vi "main.vi"() -> ()   [LabVIEW 2016]
uses:
  Common_FPGA_HealthAndStatus/DataTypes/HealthAndStatusSettings.ctl
  Common_FPGA_Modbus/DataTypes/ModbusPortSettings.ctl
  Common_FPGA_Timestamp/DataTypes/TimestampSettings.ctl
  <vilib>/Platform/TimedLoop/XDataNode/timing_clust.ctl
  <vilib>/Platform/TimedLoop/XDataNode/nitl_modes.ctl
  <vilib>/Platform/TimedLoop/XDataNode/wakeup.ctl
  <vilib>/rvi/Emulation/niFpgaGetClockAttributes.vi
  <vilib>/rvi/Emulation/niFpgaSctlEmulationGetInTimedLoop.vi
  <vilib>/rvi/Emulation/niFpgaEmulationReportErrorSimple.vi
  <vilib>/rvi/eio/common/nirviEmuTemplateMethod_errors.vi
  <vilib>/rvi/Emulation/niFpgaCriticalErrorInLSC.vi
  <vilib>/rvi/Emulation/niFpgaEmulationIsFPGAContextNoSignature.vi
  <vilib>/rvi/DataTransferAndStorage/Container/Common/niFpgaContainerGetUniqueNameForEmu.vi
  <vilib>/rvi/Memory/Memory_Emulation/niFpgaMemoryEmulationCacheClearOnFirstRun.vi
  <vilib>/rvi/Memory/Memory_Emulation/nirvimemoryEmulationManagerCache_MakeExclusive.vi
  <vilib>/rvi/Memory/Memory_Emulation/niFpgaMemoryEmulationValidateCache.vi
  <vilib>/rvi/Memory/Memory_Emulation/nirvimemoryEmulationManagerCache_InsertValue.vi
  <vilib>/Utility/error.llb/Clear Errors.vi
  <vilib>/rvi/Memory/Memory_Emulation/nirvimemoryEmulationManagerCache_ReleaseExclusive.vi
  <vilib>/rvi/Memory/Memory_Emulation/nirvimemoryEmulationManagerCache_GetValue.vi
  <vilib>/rvi/Memory/Memory_Emulation/nirvimemoryEmulationManagerCache_SetValue.vi
  <vilib>/rvi/Emulation/niFpgaProcessEmulError.vi
  <vilib>/rvi/interface/RandomDataEmulation/niFpgaRandomDataHandleErrors.vi
  <vilib>/rvi/errors/niFpgaSetErrorForExecOnDevCompSimple.vi
  <vilib>/rvi/eio/common/nirviEmuReportErrorAndStop.vi
  <vilib>/rvi/FIFO/Fifo_Resource/nirvififoEmulationSetSize.vi
  <vilib>/rvi/FIFO/Fifo_Resource/nirviFifoEmulationQueueMgr.vi
  <instcachedir>/0/nirviFifoEmulationQueueMgr_E5CAEC123FF24DC58D834DCA3CDAA9B5.lvgen/nirviFifoEmulationQueueMgr_E5CAEC123FF24DC58D834DCA3CDAA9B5_002.vi
  <vilib>/rvi/FIFO/Fifo_Resource/nirvififoEmulationDetermineInputValidOut.vi
  <vilib>/rvi/FIFO/Fifo_Resource/nirvififoEmulationCreateLock.vi
  <vilib>/rvi/FIFO/Fifo_Resource/nirvififoEmulationObtainLock.vi
  <vilib>/rvi/FIFO/Fifo_Resource/nirvififoEmulationReleaseLock.vi
  <vilib>/rvi/occurrence/nirviWaitOnOccurrenceBase.vi
  <vilib>/rvi/errors/nirviReportUnexpectedCaseInternalError.vi
  <vilib>/rvi/errors/nirviReportUnexpectedCaseInternalError (U32).vi
  <vilib>/eio/EIOMethodNode/EIOMethodNode.xnode
  <vilib>/rvi/DataTransferAndStorage/Container/XNode/niFpgaContainer.xnode
  <vilib>/rvi/DataTransferAndStorage/Register/Emulation/niFpgaRegisterEmulation.vi
  <vilib>/Platform/TimedLoop/XDataNode/XDataNode.xnode
  <vilib>/rvi/interface/RandomDataEmulation/nirviRandomDataFpgaReadWriteTemplate.vi
  <vilib>/rvi/FIFO/Fifo_Resource/nirvififoEmulationWrite.vi
  Common_FPGA_HealthAndStatus/FPGAHealthAndStatus.lvlib
  Common_FPGA_Modbus/FPGAModbus.lvlib
  Common_FPGA_Timestamp/FPGATimestamp.lvlib
  <vilib>/Platform/TimedLoop/XDataNode/XDNodeRunTimeDep.lvlib
panel:
  in  "Trigger":bool
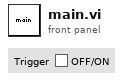
[diagram p1: front panel]
types:
  T1 = typedef "FPGATimestamp.lvlib/TimestampSettings.ctl" = cluster{"TimeRegister":refnum<k21>, "TimeSource":refnum<k21>, "IterationsPerMicrosecond":i16, "UpdateFIFO":refnum<k21>}
  T2 = typedef "FPGAModbus.lvlib/ModbusPortSettings.ctl" = cluster{"TxPort":refnum<k21>, "TxDataFIFO":refnum<k21>, "TxInternalDataFIFO":refnum<k21>, "TxHealthAndStatusFIFO":refnum<k21>, "RxPort":refnum<k21>, "RxDataFIFO":refnum<k21>, "RxHealthAndStatusFIFO":refnum<k21>, "BaseHealthAndStatusAddress":u32, "WaitForRxFrameRegister":refnum<k21>, "IRQAddress":u8, "TriggerIRQRegister":refnum<k21>, "InternalHealthAndStatusFIFO":refnum<k21>, "SoftwareControlledTrigger":refnum<k21>, "TimestampRegister":refnum<k21>, "TxTimestampFIFO":refnum<k21>}
  T3 = typedef "FPGAHealthAndStatus.lvlib/HealthAndStatusSettings.ctl" = cluster{"InternalHealthAndStatusFIFO":refnum<k21>, "HealthAndStatusQueryFIFO":refnum<k21>, "HealthAndStatusResponseFIFO":refnum<k21>, "HealthAndStatusMemory":refnum<k21>, "MemorySize":i32}
  T4 = typedef "XDNodeRunTimeDep.lvlib/timing_clust.ctl" = cluster{"Expected End [f-1]":u64, "Actual End [f-1]":u64, "Finished Late? [f-1]":bool, "Expected End [i-1]":u64, "Actual End [i-1]":u64, "Finished Late? [i-1]":bool, "Expected Start [i]":u64, "Actual Start [i]":u64, "Expected Start [f]":u64, "Actual Start [f]":u64, "Source Name":string, "Structure Name":string, "Period":i64, "Deadline":i64, "Offset":i64, "Start":i64, "Priority":i32, "Timeout":i32, "Mode":T5, "Wakeup Reason":T6, "Error":errorcluster, "Source Type":string, "Secondary Source Type":string, "Global End Time":u64, "Global Start Time":u64, "Frame Duration":u64, "Iteration Duration":u64, "Assigned CPU":i32, "I/O Scan Engine Mode":u32}
  T5 = typedef "XDNodeRunTimeDep.lvlib/nitl_modes.ctl" = enum32{"No Change", "Process missed periods, maintain original phase", "Discard missed periods, maintain original phase", "Process missed periods, ignore original phase", "Discard missed periods, ignore original phase"}
  T6 = typedef "XDNodeRunTimeDep.lvlib/wakeup.ctl" = enum32{"Normal", "Aborted", "Asynchronous wakeup", "Timing source error", "Timed loop error", "Timeout"}
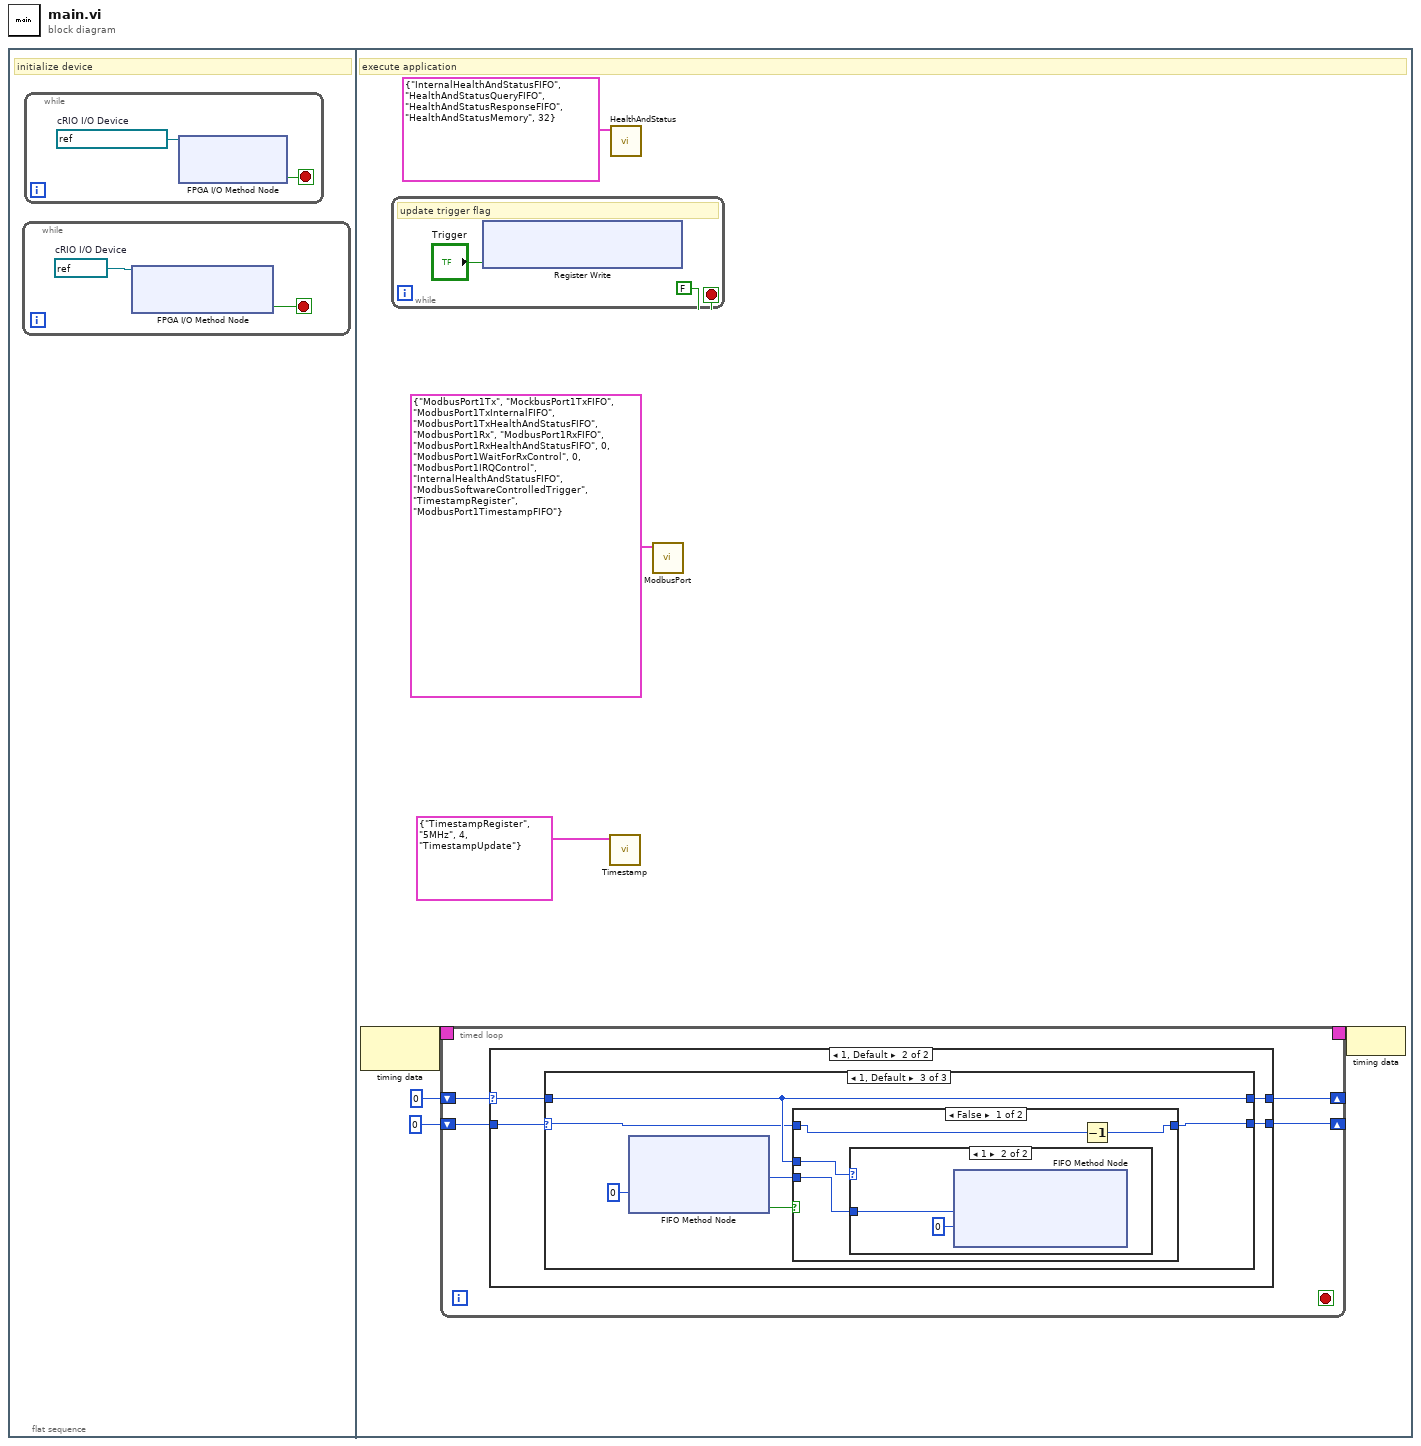
[diagram p0: block diagram]
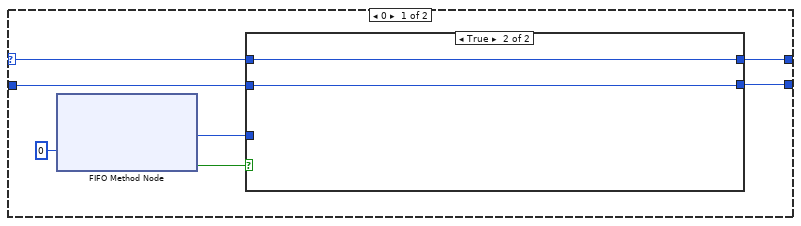
[diagram p2: hidden frame]
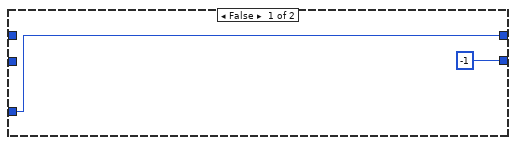
[diagram p3: hidden frame]
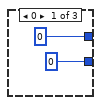
[diagram p4: hidden frame]
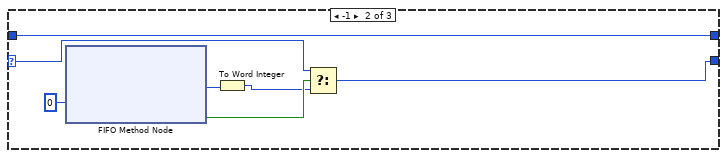
[diagram p5: hidden frame]
diagram:
  n1 = flat-sequence {
    frame #0 {
      # "initialize device"
      n2 = while {
        stop <- w1 stop-if-true
        w2 = refnum<k21> "Sync"  # cRIO I/O Device
        n3 = xnode "FPGA I/O Method Node"("FPGA I/O In"=w2) -> ("Clock Running"=w1:bool)  [unwired: 1 out]
      }
      n4 = while {
        stop <- w3 stop-if-true
        w4 = refnum<k21> "ModbusPort1-4"  # cRIO I/O Device
        n5 = xnode "FPGA I/O Method Node"("FPGA I/O In"=w4) -> ("Ready"=w3:bool)  [unwired: 1 out]
      }
    }
    frame #1 {
      # "execute application"
      n6 = node-c288() -> (w8:T4)  [unwired: 1 in]
      n7 = while {
        stop <- FALSE stop-if-true
        # "update trigger flag"
        n8 = xnode ("Register Write")("Data"="Trigger") -> ()  [unwired: 1 in, 1 out]
      }
      n9 = timed-loop {
        timing: w8 -> [_]
        timing-out: [_] -> w7
        shift-right: [w13] -> _
        shift-left: u16 0 -> [w15]
        shift-right: [w12] -> _
        shift-left: i16 0 -> [w14]
        stop <- _ stop-if-true
        n10 = case shown="1, Default" w15 {
          selector: w15 -> [w19 w27]
          tunnel: w14 -> [w16 w30]
          tunnel: [w18 w28] -> w13
          tunnel: [w17 w29] -> w12
          frame 0 {
            n11 = xnode ("FIFO Method Node")("Timeout"=0) -> ("Element"=w20:u16, "Timed Out?"=w21:bool)  [unwired: 1 in, 1 out]
            n12 = case shown="True" w21 {
              tunnel: w20 -> [w24 _]
              tunnel: w19 -> [_ w26]
              tunnel: [w24 w26] -> w18
              tunnel: [i16 -1 w25] -> w17
              tunnel: w16 -> [_ w25]
              frame False {
              }
              frame True {
              }
            }
          }
          frame 1, Default {
            n13 = case shown="1, Default" w30 {
              selector: w30 -> [_ w37 w42]
              tunnel: [i16 0 w34 w41] -> w29
              tunnel: [u16 0 w33 w44] -> w28
              tunnel: w27 -> [_ w33 w44]
              frame 0 {
              }
              frame -1 {
                n14 = xnode ("FIFO Method Node")("Timeout"=0) -> ("Element"=w36:u16, "Timed Out?"=w38:bool)  [unwired: 1 in, 1 out]
                n15 = To Word Integer(number=w36) -> (16bit integer=w35:i16)
                n16 = Select(t=w37, s=w38, f=w35) -> (s? t:f=w34:i16)
              }
              frame 1, Default {
                n17 = xnode ("FIFO Method Node")("Timeout"=0) -> ("Element"=w43:u16, "Timed Out?"=w45:bool)  [unwired: 1 in, 1 out]
                n18 = case shown="False" w45 {
                  tunnel: w44 -> [w49 _]
                  tunnel: w43 -> [w48 _]
                  tunnel: [w46 w52] -> w41
                  tunnel: w42 -> [w47 w52]
                  frame False {
                    n19 = case shown="1" w49 {
                      tunnel: w48 -> [_ w51]
                      frame 0, Default {
                      }
                      frame 1 {
                        n20 = xnode ("FIFO Method Node")("Element"=w51, "Timeout"=0) -> ()  [unwired: 1 in, 2 out]
                      }
                    }
                    n21 = Decrement(x=w47) -> (x-1=w46:i16)
                  }
                  frame True {
                  }
                }
              }
            }
          }
        }
      }
      n22 = call "Timestamp.vi"("TimestampSettings"=T1 {"TimeRegister"="TimestampRegister", "TimeSource"="5MHz", "IterationsPerMicrosecond"=4, "UpdateFIFO"="TimestampUpdate"}) -> ()  [unwired: 11 in]
      n23 = call "HealthAndStatus.vi"("HealthAndStatusSettings"=T3 {"InternalHealthAndStatusFIFO"="InternalHealthAndStatusFIFO", "HealthAndStatusQueryFIFO"="HealthAndStatusQueryFIFO", "HealthAndStatusResponseFIFO"="HealthAndStatusResponseFIFO", "HealthAndStatusMemory"="HealthAndStatusMemory", "MemorySize"=32}) -> ()  [unwired: 11 in]
      n24 = call "ModbusPort.vi"("ModbusPortSettings"=T2 {"TxPort"="ModbusPort1Tx", "TxDataFIFO"="MockbusPort1TxFIFO", "TxInternalDataFIFO"="ModbusPort1TxInternalFIFO", "TxHealthAndStatusFIFO"="ModbusPort1TxHealthAndStatusFIFO", "RxPort"="ModbusPort1Rx", "RxDataFIFO"="ModbusPort1RxFIFO", "RxHealthAndStatusFIFO"="ModbusPort1RxHealthAndStatusFIFO", "BaseHealthAndStatusAddress"=0, "WaitForRxFrameRegister"="ModbusPort1WaitForRxControl", "IRQAddress"=0, "TriggerIRQRegister"="ModbusPort1IRQControl", "InternalHealthAndStatusFIFO"="InternalHealthAndStatusFIFO", "SoftwareControlledTrigger"="ModbusSoftwareControlledTrigger", "TimestampRegister"="TimestampRegister", "TxTimestampFIFO"="ModbusPort1TimestampFIFO"}) -> ()  [unwired: 10 in]
      n25 = node-c288(w7) -> ()
    }
  }
